vi "UDPreciever.vi"() -> ()   [LabVIEW 2012]
panel:
  out "channel 11":u32[](graph)
  out "in 11":bool
  out "channel 10":u32[](graph)
  out "in 10":bool
  out "channel 9":u32[](graph)
  out "in 9":bool
  out "channel 8":u32[](graph)
  out "in 8":bool
  out "channel 7":u32[](graph)
  out "in 7":bool
  out "channel 6":u32[](graph)
  out "in 6":bool
  out "channel 5":u32[](graph)
  out "in 5":bool
  out "channel 4":u32[](graph)
  out "in 4":bool
  out "channel 3":u32[](graph)
  out "in 3":bool
  out "channel 2":u32[](graph)
  out "in 2":bool
  out "channel 1":u32[](graph)
  out "in 1":bool
  out "channel 0":u32[](graph)
  out "in 0":bool
  out "NumBins":u32
  out "Cnts/Bin":u32
  out "Prof/Hist":u32
  out "Sync":u32
  out "Channel":u32
  out "rTime":u32
  out "frameCntr":u32
  out "built packet array":string[](array[string])
  out "channel":u32
  out "built header":bool[][](array[boolean])
  out "Found Header":bool
  out "Raw Data Out":string
  out "error post-check":errorcluster
  out "End Reciever Error":errorcluster
  in  "stop reciever":bool
  out "port":u16
  out "error out post-read":errorcluster
  out "error out pre-read":errorcluster
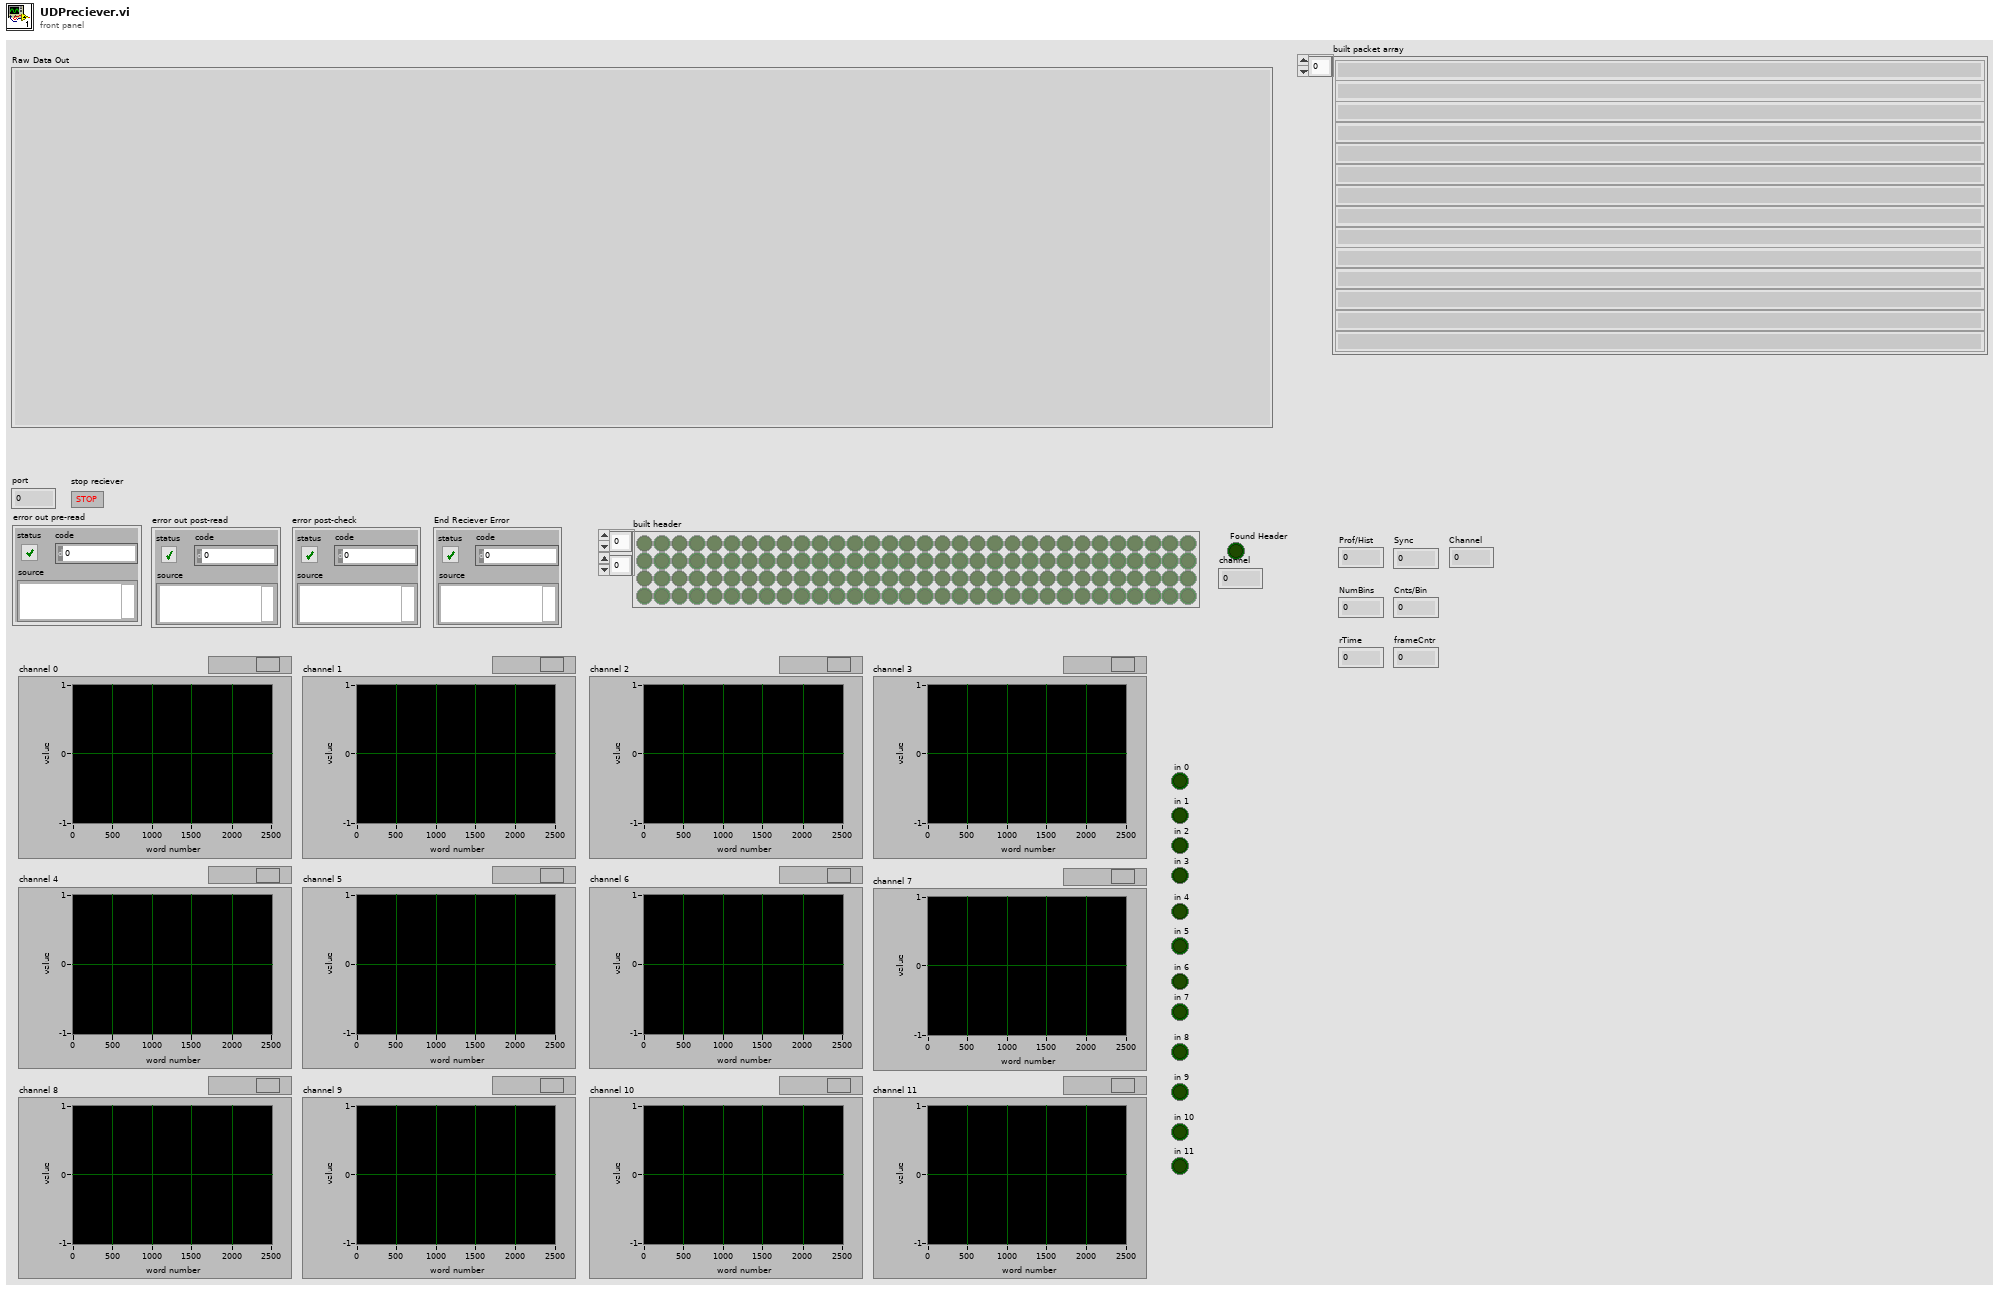
[diagram p1: front panel]
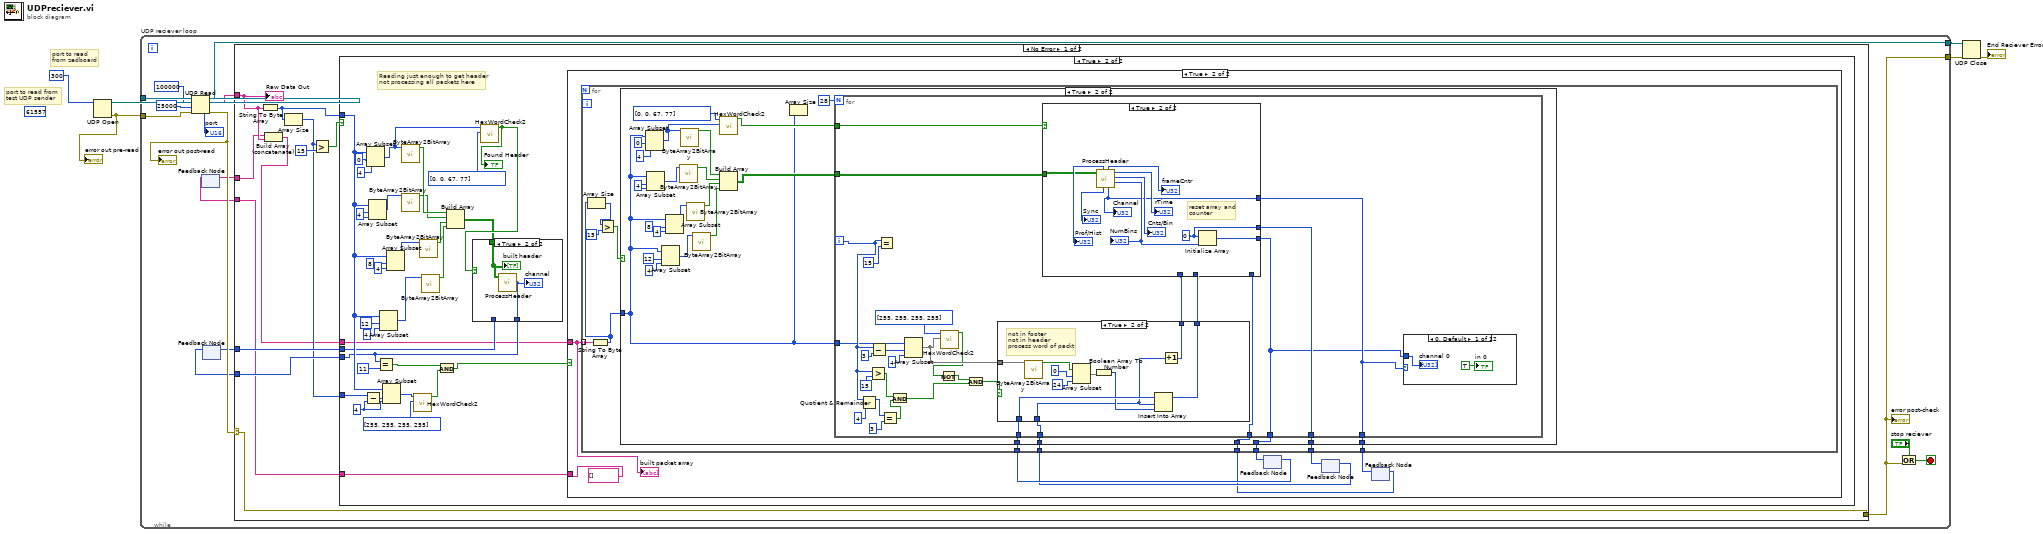
[diagram p0: block diagram]
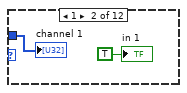
[diagram p5: hidden frame]
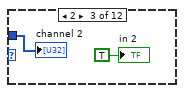
[diagram p6: hidden frame]
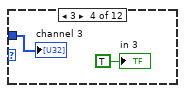
[diagram p7: hidden frame]
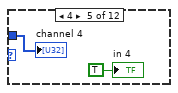
[diagram p8: hidden frame]
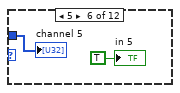
[diagram p9: hidden frame]
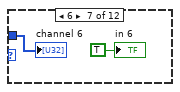
[diagram p10: hidden frame]
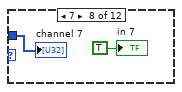
[diagram p11: hidden frame]
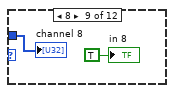
[diagram p12: hidden frame]
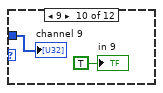
[diagram p13: hidden frame]
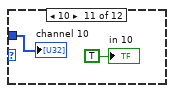
[diagram p14: hidden frame]
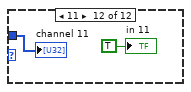
[diagram p15: hidden frame]
diagram:
  (unwired) u16 61557 ("port")
  # "port to read \nfrom zedboard"
  # "port to read from \ntest UDP sender"
  n1 = UDP Open(11:u16 300 ("port")) -> (port=w5:refnum<k16>, 0:w2:errorcluster)  [unwired: 4 in, 1 out]
  "error out pre-read" <- w2
  n2 = while "UDP reciever loop" {
    tunnel: [w21] -> w6
    tunnel: w5 -> [w20]
    tunnel: [w12] -> w4
    tunnel: w2 -> [w17]
    stop <- w19 stop-if-true
    n3 = UDP Read(connection ID=w20, max size (548)=100000, timeout ms (25000)=25000, 8:w17) -> (data out=w14:string, error out=w16:errorcluster, 3:w21:refnum<k16>, 4:→"port":u16)  [unwired: 1 out]
    "error out post-read" <- w16
    n4 = feedback #1() -> (w9:string[])  [unwired: 1 in]
    n5 = feedback #2() -> (w7:u32)  [unwired: 1 in]
    n6 = case shown="No Error" w16 {
      selector: w16 -> [w32 w198]
      tunnel: w14 -> [w31 _]
      tunnel: [w32 w198] -> w12
      tunnel: [w22 w197] -> w10
      tunnel: w9 -> [w30 w197]
      tunnel: [w27 w196] -> w8
      tunnel: w7 -> [w26 w196]
      frame No Error {
        n7 = String To Byte Array(string=w31) -> (unsigned byte array=w23:u8[])
        n8 = Build Array (concatenate)(w30, w31) -> (w24:string[])
        n9 = Array Size(array=w23) -> (size(s)=w25:i32)
        n10 = Greater?(x=w25, y=15) -> (0:w29:bool)
        n11 = case shown="True" w29 {
          tunnel: w23 -> [_ w45]
          tunnel: [w34 w38] -> w27
          tunnel: w26 -> [w34 w39]
          tunnel: w25 -> [_ w42]
          tunnel: w24 -> [w33 w36]
          tunnel: [w33 w35] -> w22
          frame False {
          }
          frame True {
            w44 = 4 ("length")
            w61 = 4 ("length")
            # "Reading just enough to get header\nnot processing all packets here"
            n12 = Subtract(x=w42, y=w44) -> (x-y=w43:i32)
            n13 = Array Subset(array=w45, index=0, length=4) -> (w50:u8[])
            n14 = Array Subset(array=w45, index=w61, length=w61) -> (w66:u8[])
            n15 = Array Subset(array=w45, index=12, length=4) -> (w48:u8[])
            n16 = Array Subset(array=w45, index=w43, length=w44) -> (w37:u8[])
            n17 = Array Subset(array=w45, index=8, length=4) -> (w65:u8[])
            n18 = call "ByteArray2BitArray.vi"("array"=w50) -> ("Array"=w56:bool[])  [unwired: 10 in]
            n19 = call "ByteArray2BitArray.vi"("array"=w66) -> ("Array"=w55:bool[])  [unwired: 10 in]
            n20 = call "HexWordCheck2.vi"("array"=u8[] [255, 255, 255, 255], "Input Array"=w37) -> ("Boolean"=w46:bool)  [unwired: 9 in]
            n21 = call "ByteArray2BitArray.vi"("array"=w65) -> ("Array"=w53:bool[])  [unwired: 10 in]
            n22 = call "ByteArray2BitArray.vi"("array"=w48) -> ("Array"=w54:bool[])  [unwired: 10 in]
            n23 = Build Array(w56, w55, w53, w54) -> (w51:bool[][])
            n24 = call "HexWordCheck2.vi"("array"=u8[] [0, 0, 67, 77], "Input Array"=w50) -> ("Boolean"=w52:bool)  [unwired: 9 in]
            "Found Header" <- w52
            n25 = case shown="True" w52 {
              tunnel: w51 -> [_ w195]
              tunnel: [w193 w194] -> w38
              tunnel: w39 -> [w193 _]
              frame False {
              }
              frame True {
                n26 = call "ProcessHeader.vi"("Array"=w195) -> ("Numeric 4"=w194:u32)  [unwired: 4 in, 6 out]
                "channel" <- w194
                "built header" <- w195
              }
            }
            n27 = Equal?(x=w38, y=u32 11) -> (x = y?=w41:bool)
            n28 = And(x=w41, y=w46) -> (x .and. y?=w47:bool)
            n29 = case shown="True" w47 {
              tunnel: w36 -> [w67 w68]
              tunnel: [w67 string[] []] -> w35
              frame False {
              }
              frame True {
                n30 = feedback #3() -> (w74:u32[])  [unwired: 1 in]
                n31 = feedback #4() -> (w72:u32)  [unwired: 1 in]
                n32 = feedback #5() -> (w70:u32)  [unwired: 1 in]
                n33 = for {
                  tunnel: w68 -> [w86] mode=indexing
                  tunnel: [w79] -> w75
                  tunnel: w74 -> [w77]
                  tunnel: [w80] -> w73
                  tunnel: w72 -> [w76]
                  tunnel: [w81] -> w71
                  tunnel: w70 -> [w78]
                  n34 = String To Byte Array(string=w86) -> (unsigned byte array=w85:u8[])
                  n35 = Array Size(array=w85) -> (size(s)=w84:i32)
                  n36 = Greater?(x=w84, y=15) -> (0:w82:bool)
                  n37 = case shown="True" w82 {
                    tunnel: w85 -> [_ w91]
                    tunnel: [w87 w99] -> w81
                    tunnel: [w88 w98] -> w80
                    tunnel: [w89 w97] -> w79
                    tunnel: w78 -> [w87 w96]
                    tunnel: w77 -> [w89 w95]
                    tunnel: w76 -> [w88 w94]
                    frame False {
                    }
                    frame True {
                      w104 = 4 ("length")
                      n38 = Array Subset(array=w91, index=0, length=4) -> (w114:u8[])
                      n39 = Array Subset(array=w91, index=w104, length=w104) -> (w100:u8[])
                      n40 = Array Subset(array=w91, index=12, length=4) -> (w113:u8[])
                      n41 = Array Subset(array=w91, index=8, length=4) -> (w101:u8[])
                      n42 = call "ByteArray2BitArray.vi"("array"=w100) -> ("Array"=w110:bool[])  [unwired: 10 in]
                      n43 = call "ByteArray2BitArray.vi"("array"=w114) -> ("Array"=w109:bool[])  [unwired: 10 in]
                      n44 = call "ByteArray2BitArray.vi"("array"=w101) -> ("Array"=w112:bool[])  [unwired: 10 in]
                      n45 = call "ByteArray2BitArray.vi"("array"=w113) -> ("Array"=w111:bool[])  [unwired: 10 in]
                      n46 = call "HexWordCheck2.vi"("array"=w114, "Input Array"=u8[] [0, 0, 67, 77] ("array")) -> ("Boolean"=w93:bool)  [unwired: 9 in]
                      n47 = Build Array(w109, w110, w112, w111) -> (w92:bool[][])
                      n48 = Array Size(array=w91) -> ()  [unwired: 1 out]
                      n49 = for {
                        N: 28 -> [_]
                        tunnel: w96 -> [w126]
                        tunnel: [w117] -> w99
                        tunnel: w94 -> [w125]
                        tunnel: [w124] -> w98
                        tunnel: [w116] -> w97
                        tunnel: w95 -> [w123]
                        tunnel: w93 -> [w120]
                        tunnel: w92 -> [w119]
                        tunnel: w91 -> [w118]
                        i -> [w127]
                        n50 = Quotient & Remainder(x=w127, y=4) -> (x-y*floor(x/y)=w139:i32)  [unwired: 1 out]
                        n51 = Greater?(x=w127, y=15 ("x")) -> (0:w141:bool)
                        n52 = Subtract(x=w127, y=3) -> (x-y=w135:i32)
                        n53 = Equal?(x=w127, y=15) -> ()  [unwired: 1 out]
                        n54 = Equal?(x=w139, y=3 ("x")) -> (x = y?=w140:bool)
                        n55 = And(x=w141, y=w140) -> (x .and. y?=w132:bool)
                        n56 = Array Subset(array=w118, index=w135, length=4) -> (w130:u8[])
                        n57 = call "HexWordCheck2.vi"("array"=w130, "Input Array"=u8[] [255, 255, 255, 255] ("array")) -> ("Boolean"=w128:bool)  [unwired: 9 in]
                        n58 = Not(x=w128) -> (.not. x?=w129:bool)
                        n59 = And(x=w129, y=w132) -> (x .and. y?=w131:bool)
                        n60 = case shown="True" w131 {
                          tunnel: w123 -> [w169 w179]
                          tunnel: w125 -> [w168 w171]
                          tunnel: w130 -> [_ w173]
                          tunnel: [w169 w172] -> w121
                          tunnel: [w168 w170] -> w122
                          frame False {
                          }
                          frame True {
                            # "not in footer \nnot in header\nprocess word of packt"
                            n61 = call "ByteArray2BitArray.vi"("array"=w173) -> ("Array"=w174:bool[])  [unwired: 10 in]
                            n62 = Array Subset(array=w174, index=0, length=24) -> (w176:bool[])
                            n63 = Boolean Array To Number(Boolean array=w176) -> (number=w175:u32)
                            n64 = Insert Into Array(array=w179, index=w171, new element=w175) -> (w172:u32[])
                            n65 = Increment(x=w171) -> (x+1=w170:u32)
                          }
                        }
                        n66 = case shown="True" w120 {
                          tunnel: w119 -> [_ w186]
                          tunnel: [w182 w185] -> w116
                          tunnel: [w181 w184] -> w124
                          tunnel: w121 -> [w182 _]
                          tunnel: w122 -> [w181 _]
                          tunnel: [w180 w183] -> w117
                          tunnel: w126 -> [w180 _]
                          frame False {
                            # "not in header, so process start of packet"
                          }
                          frame True {
                            w184 = u32 0 ("element")
                            # "reset array and \ncounter"
                            n67 = call "ProcessHeader.vi"("Array"=w186) -> ("Numeric"=w187:u32, "Numeric 7"=→"Cnts/Bin":u32, "Numeric 3"=→"rTime":u32, "Numeric 4"=w183:u32, "Numeric 2"=→"frameCntr":u32, "Numeric 5"=→"Sync":u32, "Numeric 6"=→"Prof/Hist":u32)  [unwired: 4 in]
                            "NumBins" <- w187
                            "Channel" <- w183
                            n68 = Initialize Array(w184, w187) -> (w185:u32[])
                          }
                        }
                        n69 = case shown="0, Default" w117 {
                          tunnel: w116 -> [w145 w147 w149 w151 w153 w155 w157 w159 w161 w163 w165 w167]
                          frame 0, Default {
                            "channel 0" <- w145
                            "in 0" <- TRUE ("in 11")
                          }
                          frame 1 {
                            "channel 1" <- w147
                            "in 1" <- TRUE ("in 11")
                          }
                          frame 2 {
                            "channel 2" <- w149
                            "in 2" <- TRUE ("in 11")
                          }
                          frame 3 {
                            "channel 3" <- w151
                            "in 3" <- TRUE ("in 11")
                          }
                          frame 4 {
                            "channel 4" <- w153
                            "in 4" <- TRUE ("in 11")
                          }
                          frame 5 {
                            "channel 5" <- w155
                            "in 5" <- TRUE ("in 11")
                          }
                          frame 6 {
                            "channel 6" <- w157
                            "in 6" <- TRUE ("in 11")
                          }
                          frame 7 {
                            "channel 7" <- w159
                            "in 7" <- TRUE ("in 11")
                          }
                          frame 8 {
                            "channel 8" <- w161
                            "in 8" <- TRUE ("in 11")
                          }
                          frame 9 {
                            "channel 9" <- w163
                            "in 9" <- TRUE ("in 11")
                          }
                          frame 10 {
                            "channel 10" <- w165
                            "in 10" <- TRUE ("in 11")
                          }
                          frame 11 {
                            "channel 11" <- w167
                            "in 11" <- TRUE ("in 11")
                          }
                        }
                      }
                    }
                  }
                }
                n70 = feedback-in #3(w75) -> ()
                n71 = feedback-in #4(w73) -> ()
                n72 = feedback-in #5(w71) -> ()
                "built packet array" <- w68
              }
            }
          }
        }
        "Raw Data Out" <- w31
      }
      frame Error {
      }
    }
    "error post-check" <- w12
    n73 = feedback-in #1(w10) -> ()
    n74 = feedback-in #2(w8) -> ()
    n75 = Or(x="stop reciever", y=w12) -> (x .or. y?=w19:bool)
  }
  n76 = UDP Close(connection ID=w6, 8:w4) -> (error out=→"End Reciever Error":errorcluster)  [unwired: 1 out]
